vi "young_output.vi"(0 "Output Path":path, 5 "YOUNG  Data Cluster":T1, 7 "Timestamp":dbl, 11 "Error In":errorcluster) -> (15 "Error Out":errorcluster)   [LabVIEW 2018]
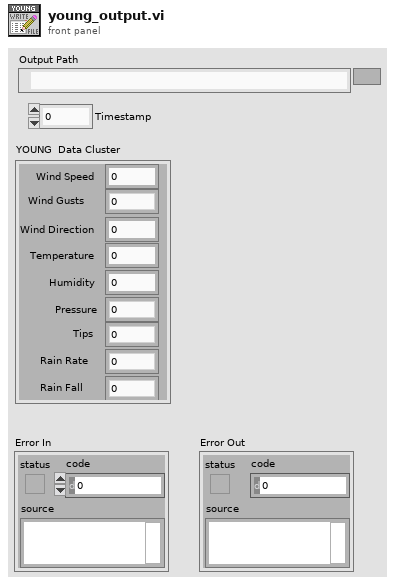
[diagram p1: front panel]
types:
  T1 = cluster{"Wind Speed":dbl, "Wind Gusts":dbl, "Wind Direction":dbl, "Temperature":dbl, "Humidity":dbl, "Pressure":dbl, "Tips":dbl, "Rain Rate":dbl, "Rain Fall":dbl}
  T2 = enum16{"open", "replace", "create", "open or create", "replace or create", "replace or create with confirmation"}
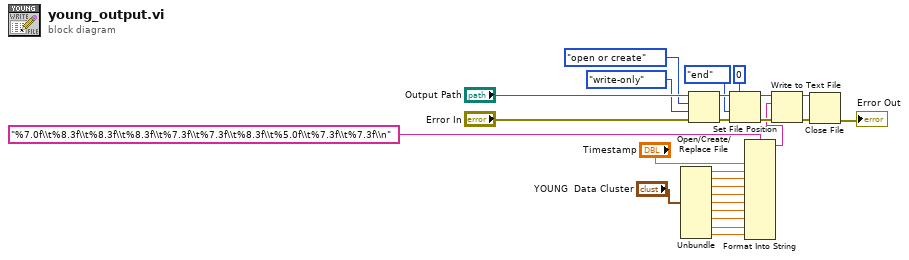
[diagram p0: block diagram]
diagram:
  n1 = Unbundle("YOUNG  Data Cluster") -> ("Wind Speed"=w9:dbl, "Wind Gusts"=w8:dbl, "Wind Direction"=w7:dbl, "Temperature"=w6:dbl, "Humidity"=w5:dbl, "Pressure"=w4:dbl, "Tips"=w3:dbl, "Rain Rate"=w2:dbl, "Rain Fall"=w1:dbl)
  n2 = Open/Create/Replace File(file path (use dialog)="Output Path", error in="Error In", operation (0:open)=T2."open or create", access (0:read/write)=enum16{"read/write", "read-only", "write-only"}."write-only") -> (refnum out=w23:refnum<file>, error out=w22:errorcluster)  [unwired: 3 out]
  n3 = Set File Position(offset (in bytes) (0)=i64 0, refnum=w23, from (0:start)=enum16{"start", "end", "current"}."end", error in=w22) -> (refnum out=w20:refnum<file>, error out=w21:errorcluster)
  n4 = Format Into String(format string="%7.0f\\t%8.3f\\t%8.3f\\t%8.3f\\t%7.3f\\t%7.3f\\t%8.3f\\t%5.0f\\t%7.3f\\t%7.3f\\n", "Timestamp", w9, w8, w7, w6, w5, w4, w3, w2, w1) -> (resulting string=w11:string)  [unwired: 2 in, 1 out]
  n5 = Write to Text File(file (use dialog)=w20, text=w11, error in=w21) -> (refnum out=w17:refnum<file>, error out=w16:errorcluster)  [unwired: 1 in, 1 out]
  n6 = Close File(refnum=w17, error in=w16) -> (error out=→"Error Out":errorcluster)  [unwired: 1 out]
